vi "Run.vi"(7 "module state":T1=enum."subpanel", 8 "error in (no error)":errorcluster, 10 "subpanel ref in":refnum<vi>, 11 "module ref in":refnum<vi>) -> (0 "error out":errorcluster, 2 "subpanel ref out":refnum<vi>, 3 "module ref out":refnum<vi>)   [LabVIEW 2019, in "Main.lvlib"]
uses:
  Main.lvlib
  State.ctl
  Framework/Tools/Tools.lvlib
panel:
  in  "window state":T2(ring)=enum."Standard"
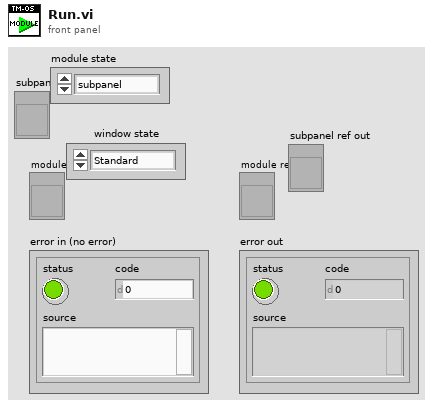
[diagram p1: front panel]
types:
  T1 = typedef "Main.lvlib/State.ctl" = enum16{"open", "closed", "subpanel"}
  T2 = enum32{"Invalid", "Standard", "Closed", "Hidden", "Minimized", "Maximized"}
  T3 = enum32{"Bad", "Idle", "Run top level", "Running"}
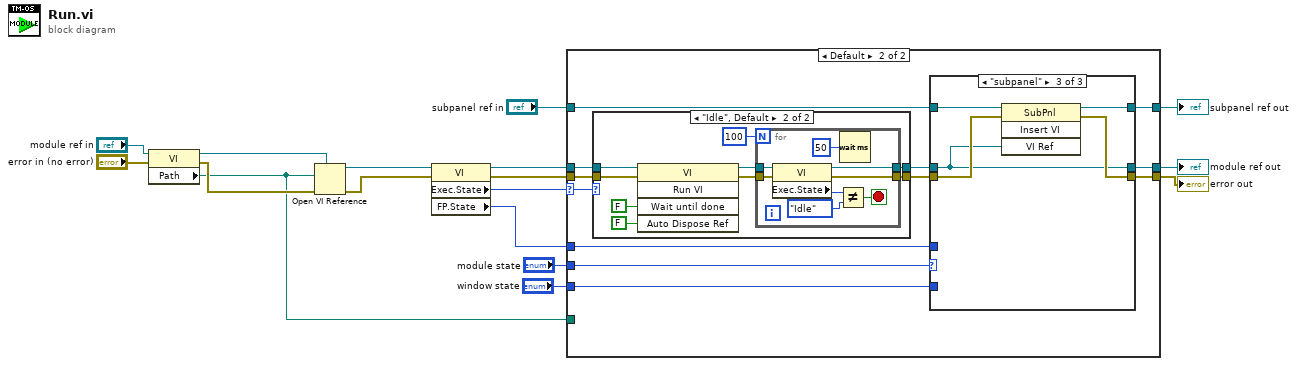
[diagram p0: block diagram]
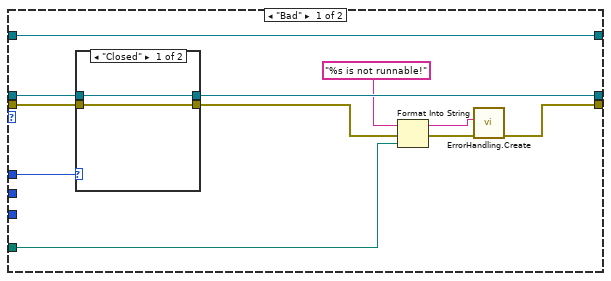
[diagram p2: hidden frame]
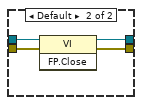
[diagram p3: hidden frame]
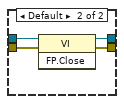
[diagram p5: hidden frame]
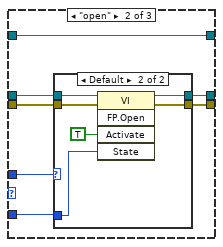
[diagram p6: hidden frame]
diagram:
  n1 = property class="VI"(reference="module ref in", error in="error in (no error)") -> (reference out=w3:refnum<vi>, error out=w17:errorcluster, "Path"=w6:path)
  n2 = Open VI Reference(type specifier VI Refnum (for type only)=w3, vi path=w6, error in (no error)=w17) -> (vi reference=w2:refnum<vi>, error out=w7:errorcluster)  [unwired: 3 in]
  n3 = property class="VI"(reference=w2, error in=w7) -> (reference out=w14:refnum<vi>, error out=w13:errorcluster, "Exec.State"=w12:T3, "FP.State"=w1:T2)
  n4 = case shown="Default" w12 {
    selector: w12 -> [_ w45]
    tunnel: [w25 w38] -> w11
    tunnel: w13 -> [w26 w46]
    tunnel: [w27 w37] -> w15
    tunnel: w14 -> [w28 w43]
    tunnel: "module state" -> [_ w44]
    tunnel: "subpanel ref in" -> [w19 w40]
    tunnel: [w19 w39] -> w9
    tunnel: w6 -> [w20 _]
    tunnel: "window state" -> [_ w36]
    tunnel: w1 -> [w18 w35]
    frame "Bad" {
      n5 = case shown="\"Closed\"" w18 {
        tunnel: w28 -> [w30 w34]
        tunnel: [w30 w33] -> w27
        tunnel: w26 -> [w29 w32]
        tunnel: [w29 w31] -> w22
        frame "Closed" {
        }
        frame Default {
          n6 = invoke class="VI" method="FP.Close"(reference=w34, error in=w32) -> (reference out=w33:refnum<vi>, error out=w31:errorcluster)  [unwired: 1 in, 1 out]
        }
      }
      n7 = Format Into String(format string="%s is not runnable!" ("explanation"), error in=w22, w20) -> (resulting string=w23:string, error out=w21:errorcluster)  [unwired: 1 in]
      n8 = call "ErrorHandling.Create.vi"("error in"=w21, "explanation"=w23) -> ("error out"=w25:errorcluster)  [unwired: 9 in]
    }
    frame Default {
      n9 = case shown="\"Idle\", Default" w45 {
        tunnel: w43 -> [w80 w89]
        tunnel: w46 -> [w79 w88]
        tunnel: [w79 w83] -> w41
        tunnel: [w80 w82] -> w42
        frame "Run top level", "Running" {
        }
        frame "Idle", Default {
          n10 = invoke class="VI" method="Run VI"(reference=w89, error in=w88, "Wait until done"=FALSE ("Wait Until Done"), "Auto Dispose Ref"=FALSE ("Auto Dispose Reference")) -> (reference out=w85:refnum<vi>, error out=w84:errorcluster)  [unwired: 1 in, 3 out]
          n11 = for {
            N: 100 -> [_]
            tunnel: w85 -> [w97]
            tunnel: w84 -> [w96]
            tunnel: [w95] -> w83
            tunnel: [w94] -> w82
            stop <- w91 stop-if-true
            n12 = property class="VI"(reference=w97, error in=w96) -> (reference out=w94:refnum<vi>, error out=w95:errorcluster, "Exec.State"=w93:T3)
            n13 = Not Equal?(x=w93, y=T3."Idle" ("Execution:State")) -> (x != y?=w91:bool)
            n14 = Wait (ms)(milliseconds to wait=u32 50) -> ()  [unwired: 1 out]
          }
        }
      }
      n15 = case shown="\"subpanel\"" w44 {
        tunnel: w42 -> [w49 w60 w74]
        tunnel: w41 -> [w48 w65 w76]
        tunnel: [w51 w64 w74] -> w37
        tunnel: [w50 w63 w75] -> w38
        tunnel: w40 -> [w52 w62 w78]
        tunnel: [w52 w62 w77] -> w39
        tunnel: w36 -> [_ w61 _]
        tunnel: w35 -> [w47 w59 _]
        frame "closed" {
          n16 = case shown="\"Closed\"" w47 {
            tunnel: [w54 w58] -> w51
            tunnel: [w53 w57] -> w50
            tunnel: w49 -> [w54 w56]
            tunnel: w48 -> [w53 w55]
            frame "Closed" {
            }
            frame Default {
              n17 = invoke class="VI" method="FP.Close"(reference=w56, error in=w55) -> (reference out=w58:refnum<vi>, error out=w57:errorcluster)  [unwired: 1 in, 1 out]
            }
          }
        }
        frame "open" {
          n18 = case shown="Default" w59 {
            tunnel: w65 -> [w66 w73]
            tunnel: [w67 w72] -> w64
            tunnel: [w66 w71] -> w63
            tunnel: w61 -> [_ w69]
            tunnel: w60 -> [w67 w68]
            frame "Standard" {
            }
            frame Default {
              n19 = invoke class="VI" method="FP.Open"(reference=w68, error in=w73, "Activate"=TRUE ("Activate?"), "State"=w69) -> (reference out=w72:refnum<vi>, error out=w71:errorcluster)  [unwired: 1 in, 3 out]
            }
          }
        }
        frame "subpanel" {
          n20 = invoke on="Invoke Node" class="SubPnl" method="Insert VI"(reference=w78, error in=w76, "VI Ref"=w74) -> (reference out=w77:refnum<vi>, error out=w75:errorcluster)  [unwired: 1 in, 2 out]
        }
      }
    }
  }
  "error out" <- w11
  "module ref out" <- w15
  "subpanel ref out" <- w9
